vi "Battery_scale.vi"() -> ()   [LabVIEW 2014]
panel:
  out "Battery_Scale":dbl
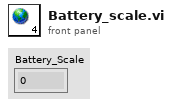
[diagram p1: front panel]
diagram:
